vi "setGainByPSSN.vi"(8 "error in (no error)":errorcluster, 9 "Sensor Name":string[](array[string])=["R44 _S00", "R04_S20", "R00_S22", "R40_S02"], 10 "PSSN":dbl[](array[numeric]), 11 "ZTAAC in":refnum<class "ZTAAC.lvclass">) -> (0 "error out":errorcluster, 3 "ZTAAC out":refnum<class "ZTAAC.lvclass">)   [LabVIEW 2016, in "OfcFunc.lvlib" / "ZTAAC.lvclass"]
doc: "Set the gain value based on the normalized point spread function (PSSN)."
uses:
  ZTAAC.lvclass
  ZTAAC.lvclass/ZTAAC.ctl
  OptStateEsti/OptStateEsti.lvclass
  OptCtrl/OptCtrl.lvclass
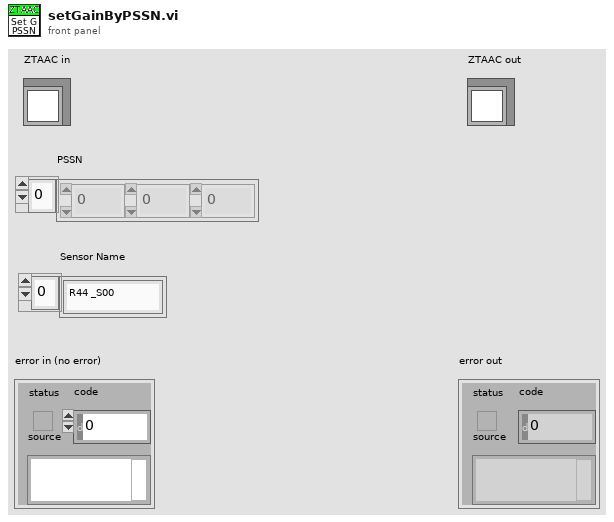
[diagram p1: front panel]
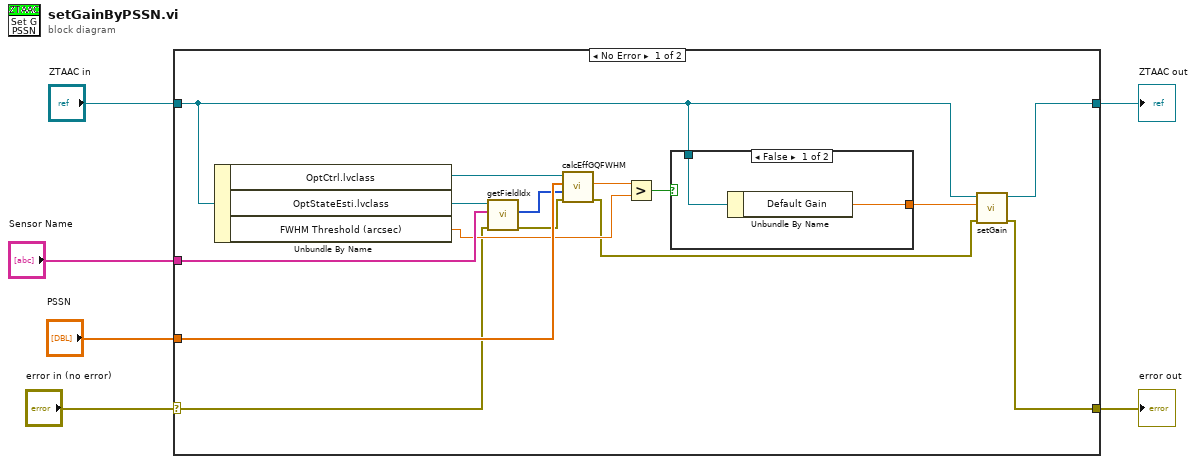
[diagram p0: block diagram]
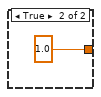
[diagram p2: hidden frame]
diagram:
  n1 = case shown="No Error" "error in (no error)" {
    selector: "error in (no error)" -> [w10 w26]
    tunnel: [w7 w26] -> w5
    tunnel: [w11 w25] -> w3
    tunnel: "ZTAAC in" -> [w13 w25]
    tunnel: "Sensor Name" -> [w20 _]
    tunnel: "PSSN" -> [w18 _]
    frame No Error {
      n2 = Unbundle By Name(w13) -> ("OptCtrl.lvclass"=w19:refnum<class "OptCtrl.lvclass">, "OptStateEsti.lvclass"=w21:refnum<class "OptStateEsti.lvclass">, "FWHM Threshold (arcsec)"=w15:dbl)
      n3 = call "getFieldIdx.vi"("error in (no error)"=w10, "Sensor Name"=w20, "OptStateEsti in"=w21) -> ("error out"=w9:errorcluster, "Field Idx"=w17:i32[])  [unwired: 6 in, 1 out]
      n4 = call "calcEffGQFWHM.vi"("error in (no error)"=w9, "Field Idx"=w17, "PSSN"=w18, "OptCtrl in"=w19) -> ("error out"=w8:errorcluster, "Effective GQFWHM (arcsec)"=w16:dbl)  [unwired: 5 in, 1 out]
      n5 = Greater?(x=w16, y=w15) -> (0:w14:bool)
      n6 = case shown="False" w14 {
        tunnel: w13 -> [w23 _]
        tunnel: [w22 1.0 ("Default Gain")] -> w12
        frame False {
          n7 = Unbundle By Name(w23) -> ("Default Gain"=w22:dbl)
        }
        frame True {
        }
      }
      n8 = call "setGain.vi"("error in (no error)"=w8, "Gain"=w12, "ZTAAC in"=w13) -> ("error out"=w7:errorcluster, "ZTAAC out"=w11:refnum<class "ZTAAC.lvclass">)  [unwired: 7 in]
    }
    frame Error {
    }
  }
  "error out" <- w5
  "ZTAAC out" <- w3
